vi "Reader and writer.vi"() -> ()   [LabVIEW 2014]
panel:
  out "error out 2":errorcluster
  out "Array":dbl[][](array[numeric])
  in  "SEND DATA":bool
  out "data out":dbl[][](array[numeric])
  in  "stop 2":bool
  out "error out":errorcluster
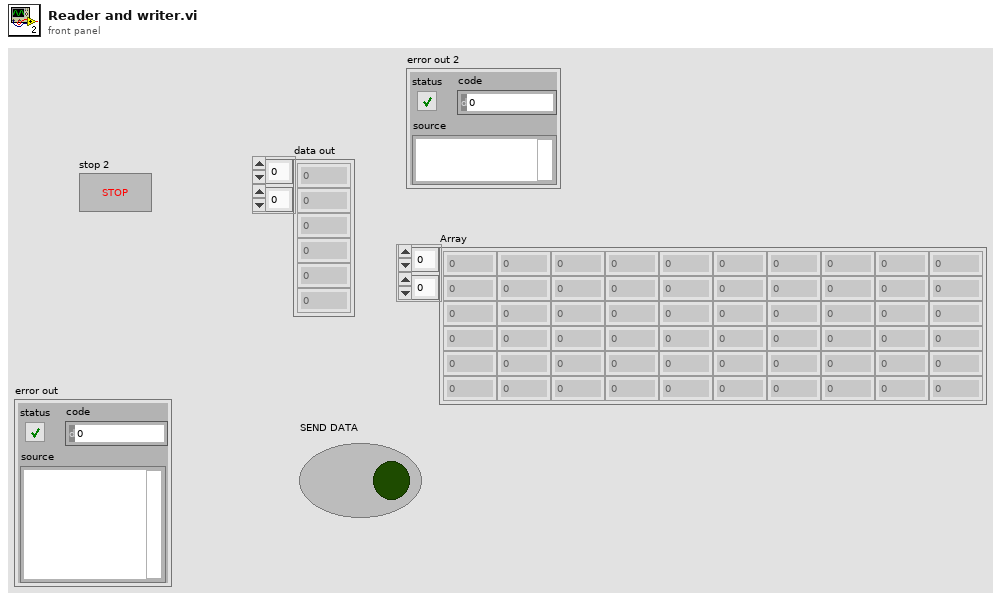
[diagram p1: front panel]
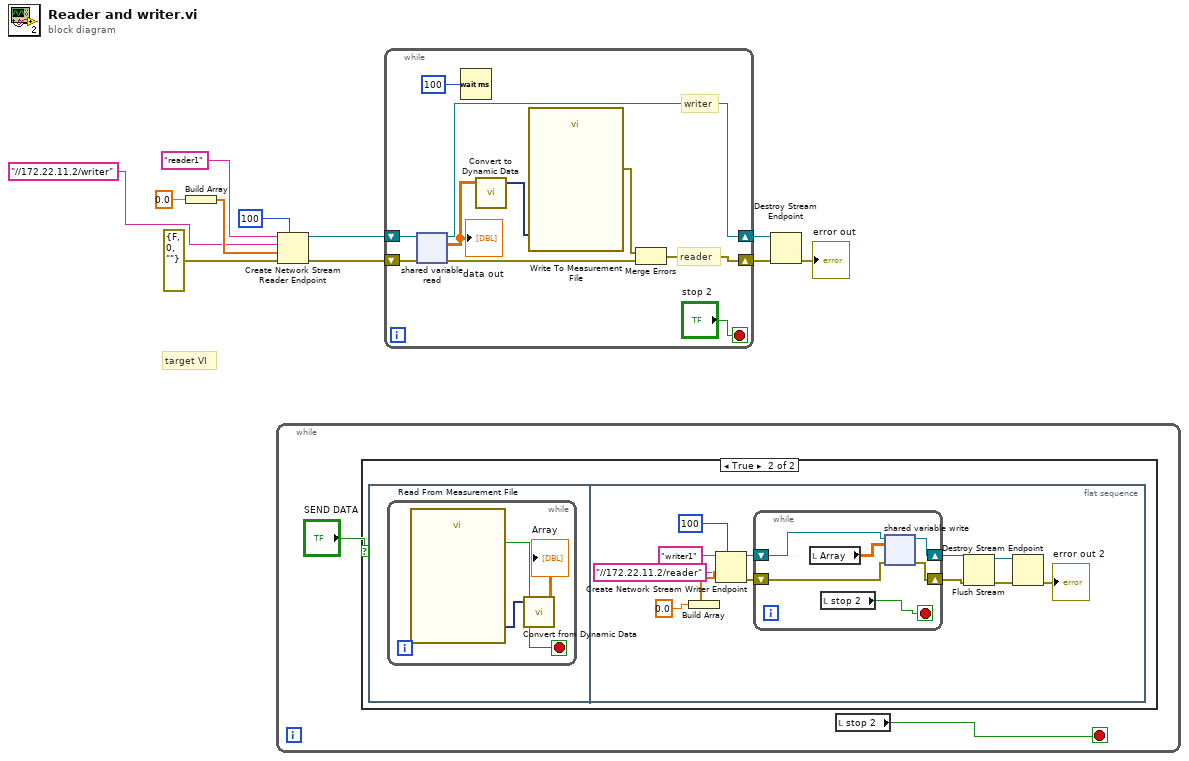
[diagram p0: block diagram]
diagram:
  # "target VI"
  n1 = Build Array(0.0) -> (w5:dbl[])
  n2 = while {
    stop <- w13 stop-if-true
    n3 = case shown="True" "SEND DATA" {
      frame False {
      }
      frame True {
        n4 = flat-sequence {
          frame #0 {
            n5 = while {
              stop <- w14 stop-if-true
              n6 = call "Read From Measurement File"() -> ("Signals"=w16:dynamicdata, "EOF?"=w14:bool)  [unwired: 6 in, 4 out]
              n7 = call "Convert from Dynamic Data"("Dynamic Data Type"=w16) -> ("Array"=→"Array":dbl[][])  [unwired: 3 in]
            }
          }
          frame #1 {
            n8 = Build Array(0.0) -> (w26:dbl[])
            n9 = Create Network Stream Writer Endpoint(7:100 ("writer buffer size"), 9:w26, 10:"//172.22.11.2/reader" ("reader url"), 11:"writer1" ("writer name")) -> (0:w24:errorcluster, 3:w25:refnum<k21>)  [unwired: 3 in]
            n10 = while {
              shift-right: [w31] -> w22
              shift-left: w24 -> [w33]
              shift-right: [w32] -> w23
              shift-left: w25 -> [w34]
              stop <- w29 stop-if-true
              n11 = local read "Array"() -> (w30:dbl[][])
              n12 = local read "stop 2"() -> (w29:bool)
              n13 = shared-variable-write(w34, w33, w30) -> (w32:refnum<k21>, w31:errorcluster)  [unwired: 1 in, 1 out]
            }
            n14 = Flush Stream(8:w22, 11:w23) -> (0:w21:errorcluster, 3:w20:refnum<k21>)  [unwired: 2 in, 1 out]
            n15 = Destroy Stream Endpoint(8:w21, 11:w20) -> (0:→"error out 2":errorcluster)
          }
        }
      }
    }
    n16 = local read "stop 2"() -> (w13:bool)
  }
  n17 = Create Network Stream Reader Endpoint(7:100 ("reader buffer size"), 8:errorcluster {"status"=FALSE, "code"=0, "source"=""} ("error in (no error)"), 9:w5, 10:"//172.22.11.2/writer" ("writer url"), 11:"reader1" ("writer name")) -> (0:w8:errorcluster, 3:w9:refnum<k21>)  [unwired: 2 in]
  n18 = while {
    shift-right: [w37] -> w4
    shift-left: w9 -> [w36]
    shift-right: [w38] -> w3
    shift-left: w8 -> [w35]
    stop <- "stop 2" stop-if-true
    # "writer"
    # "reader"
    n19 = shared-variable-read(w36, w35) -> (w37:refnum<k21>, w42:errorcluster, w39:dbl[][])  [unwired: 2 in, 1 out]
    "data out" <- w39
    n20 = Wait (ms)(milliseconds to wait=u32 100) -> ()  [unwired: 1 out]
    n21 = call "Convert to Dynamic Data"("2D Array"=w39) -> ("Dynamic Data Type"=w40:dynamicdata)  [unwired: 3 in]
    n22 = call "Write To Measurement File"("Signals"=w40) -> ("error out"=w43:errorcluster)  [unwired: 16 in, 2 out]
    n23 = Merge Errors(w43, w42) -> (w38:errorcluster)
  }
  n24 = Destroy Stream Endpoint(8:w3, 11:w4) -> (0:→"error out":errorcluster)
